vi "Name plot legend from array.vi"(4 "Force write (F)":bool, 6 "Enabled (1-10)(1)":u32=1, 7 "Names legend":string[](array[string]), 8 "error in (no error)":errorcluster, 11 "Chart in":refnum<vi>) -> (0 "error out":errorcluster)   [LabVIEW 2013]
doc: "Names legend of chart from array\nif number of elements in array is 1..10 or force write input is true\nadjusts the number of rows in legend and disables scrollbars"
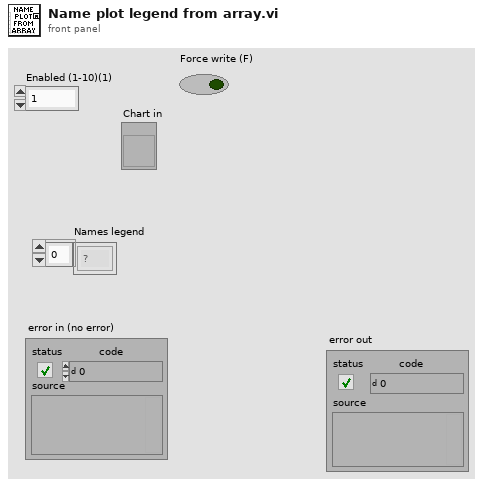
[diagram p1: front panel]
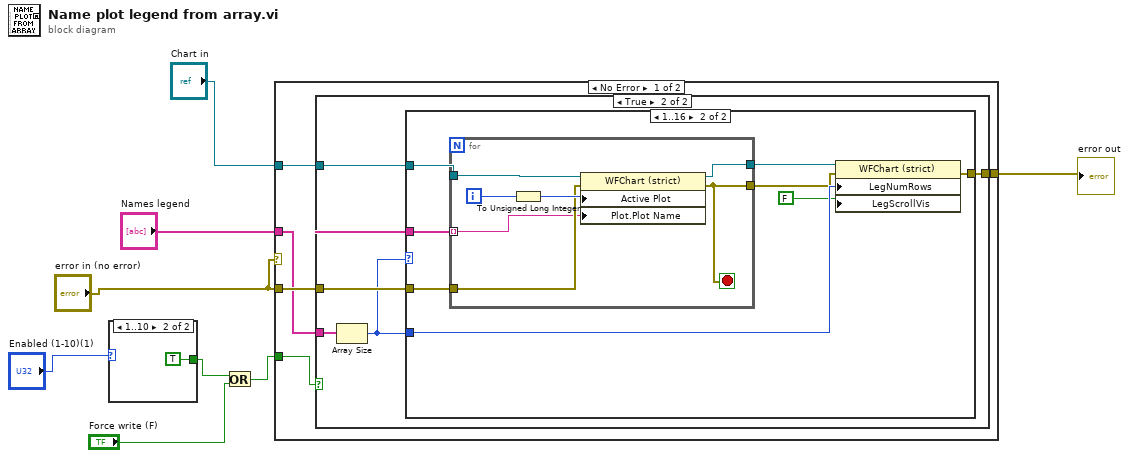
[diagram p0: block diagram]
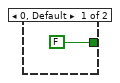
[diagram p2: hidden frame]
diagram:
  n1 = case shown="1..10" "Enabled (1-10)(1)" {
    tunnel: [FALSE TRUE] -> w3
    frame 0, Default {
    }
    frame 1..10 {
    }
  }
  n2 = Or(x=w3, y="Force write (F)") -> (x .or. y?=w2:bool)
  n3 = case shown="No Error" "error in (no error)" {
    tunnel: "Chart in" -> [w15 _]
    tunnel: "error in (no error)" -> [w14 w38]
    tunnel: "Names legend" -> [w13 _]
    tunnel: [w12 w38] -> w5
    tunnel: w2 -> [w11 _]
    frame No Error {
      n4 = case shown="True" w11 {
        tunnel: w15 -> [_ w21]
        tunnel: w14 -> [w16 w20]
        tunnel: w13 -> [_ w19]
        tunnel: [w16 w18] -> w12
        frame False {
        }
        frame True {
          n5 = Array Size(array=w19) -> (size(s)=w17:i32)
          n6 = case shown="1..16" w17 {
            tunnel: w21 -> [_ w30]
            tunnel: w20 -> [w22 w29]
            tunnel: w19 -> [_ w28]
            tunnel: w17 -> [_ w27]
            tunnel: [w22 w24] -> w18
            frame 0, Default {
            }
            frame 1..16 {
              n7 = for {
                tunnel: w30 -> [w37]
                tunnel: w29 -> [w34]
                tunnel: w28 -> [w33] mode=indexing
                tunnel: [w32] -> w26
                tunnel: [w31] -> w23
                i -> [w36]
                stop <- w32 stop-if-true
                n8 = To Unsigned Long Integer(number=w36) -> (unsigned 32bit integer=w35:u32)
                n9 = property class="WFChart (strict)"(reference=w37, error in=w34, "Active Plot"=w35, "Plot.Plot Name"=w33) -> (reference out=w31:refnum<vi>, error out=w32:errorcluster)
              }
              n10 = property class="WFChart (strict)"(reference=w23, error in=w26, "LegNumRows"=w27, "LegScrollVis"=FALSE ("Legend:Scrollbar Visible")) -> (error out=w24:errorcluster)  [unwired: 1 out]
            }
          }
        }
      }
    }
    frame Error {
    }
  }
  "error out" <- w5
